vi "VIRef_Get Parent.vi"(8 "Error":errorcluster, 9 "Get Ref? (t)":bool=TRUE, 11 "Generations Back (1:parent)":i32=1) -> (0 "Error Out":errorcluster, 1 "Call Chain Out":string[](array[string]), 2 "Parent Vi Name Out":string, 3 "VI Refnum Out":refnum<vi>)   [LabVIEW 2023]
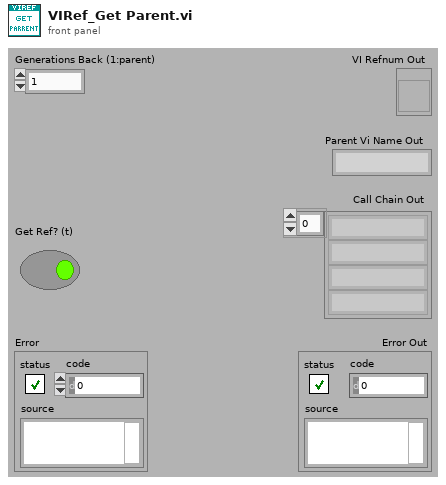
[diagram p1: front panel]
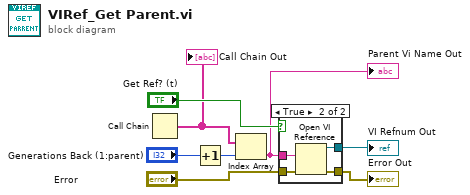
[diagram p0: block diagram]
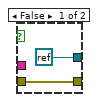
[diagram p2: hidden frame]
diagram:
  n1 = Call Chain() -> (call chain=w4:string[])
  "Call Chain Out" <- w4
  n2 = Increment(x="Generations Back (1:parent)") -> (x+1=w1:i32)
  n3 = Index Array(array=w4, index=w1) -> (element=w6:string)
  "Parent Vi Name Out" <- w6
  n4 = case shown="True" "Get Ref? (t)" {
    tunnel: [refnum<k0> refnum w14] -> w2
    tunnel: [w9 w13] -> w3
    tunnel: w6 -> [_ w12]
    tunnel: "Error" -> [w9 w11]
    frame False {
    }
    frame True {
      n5 = Open VI Reference(vi path=w12, error in (no error)=w11) -> (vi reference=w14:refnum<vi>, error out=w13:errorcluster)  [unwired: 4 out]
    }
  }
  "Error Out" <- w3
  "VI Refnum Out" <- w2
